vi "Create module message.vi"(7 "ID":string, 8 "error in (no error)":errorcluster, 9 "method":string, 10 "module":string, 11 "params":variant) -> (0 "error out":errorcluster, 3 "message data":variant)   [LabVIEW 2020]
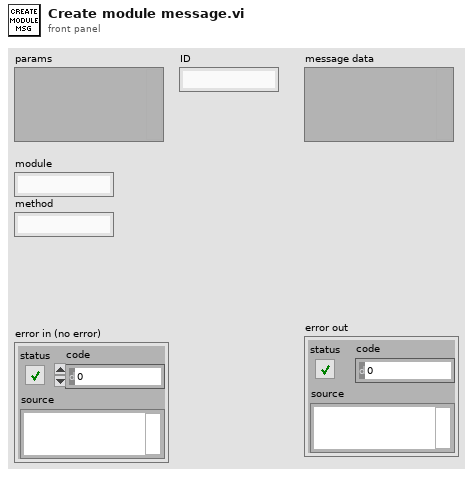
[diagram p1: front panel]
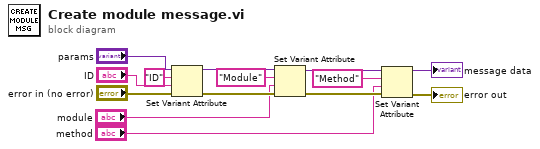
[diagram p0: block diagram]
diagram:
  n1 = Set Variant Attribute(Variant="params", name="ID", value="ID", error in="error in (no error)") -> (Variant out=w11:variant, error out=w12:errorcluster)  [unwired: 1 out]
  n2 = Set Variant Attribute(Variant=w11, name="Module", value="module", error in=w12) -> (Variant out=w4:variant, error out=w8:errorcluster)  [unwired: 1 out]
  n3 = Set Variant Attribute(Variant=w4, name="Method", value="method", error in=w8) -> (Variant out=→"message data":variant, error out=→"error out":errorcluster)  [unwired: 1 out]
